vi "Dichtheitstest.vi"() -> ()   [LabVIEW 2020, in "Erweiterte Konfig.lvlib"]
uses:
  Erweiterte Konfig.lvlib
  Visualisierungs Elemente/Button.ctl
  Visualisierungs Elemente/Zahlen-Ausgabefeld.ctl
  Dichtheitstest Umfang.ctl
  Funktionstasten/Freigabe Aktionen.ctl
  PNS/Aktionen FGV Grenzwerte.ctl
  FGV PID Aktionen.ctl
  Aktionen Dichtheitstest.ctl
  Stoerungen/Stoerungen Messgeraet/Aktionen Kommunikation Stoerung.ctl
  Status Dichtheitstest Aktionen.ctl
  Funktionstasten/Funktionstasten-Aktion.ctl
  Funktionstasten/Zustaende.ctl
  Schedule Modul/Aktion FGV Testdaten sammeln.ctl
  Amium PNS/AK Kommunikation/Amium Kommandos verwalten Aktionen.ctl
  SysLog/SysLog Interface.ctl
  Stoerungen/Stoerungen.lvlib
  Funktionstasten/Funktionstasten.lvlib
  Allgemein/allgemeine Sub-VIs.lvlib
  cRIO/PC/Kommunikation mit cRIO.lvlib
  Sprachverwaltung/Sprachverwaltung.lvlib
  SysLog/SysLog.lvlib
  Amium PNS/AK Kommunikation/AK Kommunikation.lvlib
  Auto Kalibrieren/VI Auto Kalibrieren.vi
  Auto Kalibrieren/Auto Kalibrieren.lvlib
  PNS/PNS.lvlib
  Schedule Modul/Schedule Modul.lvlib
  Sprachverwaltung/FGV Aktion Tabelle zerlegen.ctl
panel:
  out "Dichtheitstest Umfang":T1 items=["Pumpe / Filter / FT-IR / PNS", "Pumpe / Filter / FT-IR", "Filter / FT-IR", "FT-IR"]
  out "Status":string
  out "Druckanstieg:":T2
  out "Verstrichene Zeit:":T2
  out "Zeitdauer:":T2
  out "max. Anstieg:":T2 caption="max. Druckanstieg:"
  out "Druck FT-IR:":T2 format="%.3f"
  in  "BEENDEN":T3
  # "Dichtheitstest"
  # "bar"
  # "mbar"
  # "mbar"
  # "sec"
  # "sec"
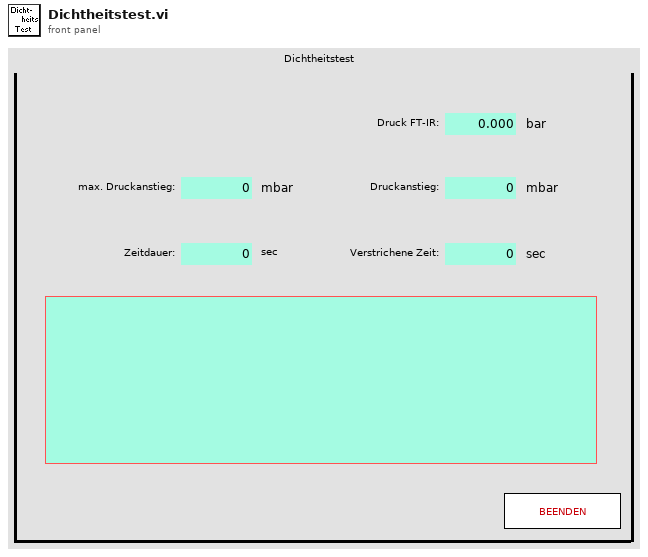
[diagram p1: front panel]
types:
  T1 = typedef "Erweiterte Konfig.lvlib/Dichtheitstest Umfang.ctl" = u16
  T2 = typedef "Zahlen-Ausgabefeld.ctl" = sgl
  T3 = typedef "Button.ctl" = bool
  T4 = typedef "PNS.lvlib/Aktionen FGV Grenzwerte.ctl" = enum16{"lesen", "Grenzw. schreiben", "Anweisungscode", "IP-Adresse", "laden", "speichern", "Anweisungscode vorgeben"}
  T5 = typedef "Funktionstasten.lvlib/Freigabe Aktionen.ctl" = enum16{"prüfen", "Freigabe?", "lesen"}
  T6 = typedef "Erweiterte Konfig.lvlib/Status Dichtheitstest Aktionen.ctl" = enum16{"lesen", "Zeitstempel", "Daten", "läuft", "Protokolldaten"}
  T7 = typedef "Stoerungen.lvlib/Aktionen Kommunikation Stoerung.ctl" = enum16{"lesen", "init", "FT-IR Komm", "FT-IR Betriebsart", "FT-IR Hintergrund", "cRIO Komm", "PNS Komm", "Dichtheitstest", "Life Bit", "FTIR Komm AK", "PMA Komm", "FID Komm", "PMA Cal", "FID Ch4 Cal", "FID THC Cal", "Cal Timeout", "VFS 1 Komm", "VFS 2 Komm", "VFS 3 Komm", "VFS 4 Komm", "TRE 08 Komm", "CG-Test vorzeitig", "CG-Test Span 1", "CG-Test Span 2", "CG-Test Span 3", "CG-Test Messgas", "CG-Test löschen", "Test", "Amium AK", "AK Recept konfig", "AK Name konfig", "AK EKFG konfig"}
  T8 = typedef "Erweiterte Konfig.lvlib/FGV PID Aktionen.ctl" = enum16{"Lesen", "Schreiben PID", "Schreiben Sonstige", "Dichtheitstest", "Aktionen Dicht.", "Parameter Sensor"}
  T9 = typedef "Erweiterte Konfig.lvlib/Aktionen Dichtheitstest.ctl" = enum16{"Initialisieren", "Unterdruck aufbauen", "Prop schließen", "Warten", "Auswertung", "Fertig"}
  T10 = typedef "Steuerung PNS.lvclass/Anlegengrenzwerte PNS.ctl" = cluster{"Filter:":T11, "Ventilplatte:":T11, "Heizleitung 1:":T11, "Heizleitung 2:":T11, "Heizleitung 3:":T11, "Heizleitung 4:":T11, "Heizleitung 5:":T11, "Heizleitung 6:":T11}
  T11 = typedef "Steuerung PNS.lvclass/Anlagengrenzwerte Parameteranzeige.ctl" = cluster{"Sollwert":T12, "Warn-Min":T12, "Warn-Max":T12, "Abschalt-Min":T12, "Abschalt-Max":T12, "Regler":u16, "AnlagenParameter":string}
  T12 = typedef "Zahlen-Eingabefeld.ctl" = sgl
  T13 = typedef "Erweiterte Konfig.lvlib/Sonstige Parameter.ctl" = cluster{"Lüfter langsam":sgl, "Lüfter schnell":sgl, "FT-IR Kühlung Soll":sgl, "FT-IR Kühlung Max":sgl, "Überwachung":T14, "Befüllung aktiv":T15, "Stickstoff Befüllzeit":sgl, "Befüllintervall":sgl, "Kalibrierwert FT-IR":sgl, "Offset Ausgang":sgl, "Offset FT-IR":sgl, "Offset Druck FT-IR":sgl, "Dichtheitstest Zeit":sgl, "Dichtheitstest Abfall":sgl, "Dichtheitstest Umfang":T1, "Offset Umgebung":sgl, "Max Taupunkt":sgl, "Pumpendrehzahl":sgl, "ext. Befüllung":T15, "Ext. Stickstoff Befüllzeit":sgl}
  T14 = typedef "Auswahlfeld.ctl" = u16
  T15 = typedef "LogKonfig.lvlib/Auswahlfeld aktiviert-deaktiviert.ctl" = u16
  T16 = typedef "Verwaltung - cRIO.lvlib/Analog Eingaenge.ctl" = cluster{"AI0: Durchfluss FT-IR":sgl, "AI1: Druck Ausgang":sgl, "AI2: Umgebungsdruck":sgl, "AI3: Druck FT-IR":sgl, "AI4: Druck CalGas":sgl, "AI5: Reserve":sgl, "AI6: Reserve":sgl, "AI7: Reserve":sgl, "Rohwert Durchfluss FT-IR":sgl, "Rohwert Druck Ausgang":sgl, "Rohwert Umgebungsdruck":sgl, "Rohwert Druck FT-IR":sgl, "Rohwert Druck CalGas":sgl, "Rohwert AI5":sgl, "Rohwert AI6":sgl, "Rohwert AI7":sgl, "Rohwert Diffdruck mbar FTIR":sgl}
  T17 = typedef "Erweiterte Konfig.lvlib/Dichtheitstest Protokoll.ctl" = cluster{"Startzeit":timestamp, "Endzeit":timestamp, "Startdruck":sgl, "Enddruck":sgl, "Dichtheitstest Umfang":T1}
  T18 = typedef "Schedule Modul.lvlib/Aktion FGV Testdaten sammeln.ctl" = enum16{"lesen", "Dichtheitstest", "CalGasTest", "T90", "Kalibrieren", "init", "Kalender Daten"}
  T19 = typedef "Funktionstasten.lvlib/Zustaende.ctl" = enum16{"Standby", "Pause", "Eco", "Messen", "Kalibrieren", "Spülen Filter", "Spülen Leitung", "Umgebungsluft", "0-Gas", "Cal-Gas", "CG zu PNS", "-------------", "Init 1", "Init 2", "Init 3", "Init 4", "Messen vorbereiten", "Messen durchführen", "Exit"}
  T20 = typedef "Funktionstasten.lvlib/Funktionstasten-Aktion.ctl" = enum16{"Initialisieren", "Zustand setzen", "Taste gedrückt", "Fehler speichern", "Lesen", "Manuell", "Remote", "Bitparallel", "Samplepoint", "Zeit Prüfen", "reset Umschalten"}
  T21 = typedef "Schedule Modul.lvlib/Ergebnis Dichtheitstest.ctl" = cluster{"Druck FT-IR:":T2, "max. Anstieg:":T2, "Druckanstieg:":T2, "Zeitdauer:":T2, "Verstrichene Zeit:":T2, "Fehler":bool, "Unterdruck nicht erreicht ":bool}
  T22 = typedef "Amium PNS.lvlib/AK Kommunikation.lvlib/Amium Kommandos verwalten Aktionen.ctl" = enum16{"lesen", "setzen Ende", "setzen Pos1", "senden", "initalisieren", "prüfen", "Kommandos"}
  T23 = typedef "Sprachverwaltung.lvlib/FGV Aktion Tabelle zerlegen.ctl" = enum16{"laden", "vereinzeln", "speichern"}
  T24 = typedef "SysLog.lvlib/SysLog Interface.ctl" = cluster{"FehlermeldungsCode":i32, "ErfolgsmeldungsCode":i32, "ParameterListenString":string, "Anzeige":bool, "SysLogIcon":enum16{"OK", "Warnung", "Fehler"}, "intern":bool}
  T25 = typedef "Stoerungen.lvlib/Stoerungen Messgeraete.ctl" = cluster{"FT-IR Komm":bool, "FT-IR Betriebsart":bool, "FT-IR Hintergrundscan":bool, "Dichtheitstest":bool, "cRIO Komm":bool, "PNS Komm":bool, "Life Bit":bool, "FT-IR AK Komm":bool, "PMA Komm":bool, "FID Komm":bool, "PMA Cal":bool, "FID CH4 Cal":bool, "FID THC Cal":bool, "Cal Timeout":bool, "VFS 1 Komm":bool, "VFS 2 Komm":bool, "VFS 3 Komm":bool, "VFS 4 Komm":bool, "TRE 08 Komm":bool, "CG-Test":bool, "CG-Test 1":bool, "CG-Test 2":bool, "CG-Test 3":bool, "Messgas - Eingang":bool, "Amium AK Komm":bool, "AK Rezept nicht konfiguriert ":bool, "AK Name nicht konfiguriert":bool, "AK EKFG nicht konfiguriert":bool}
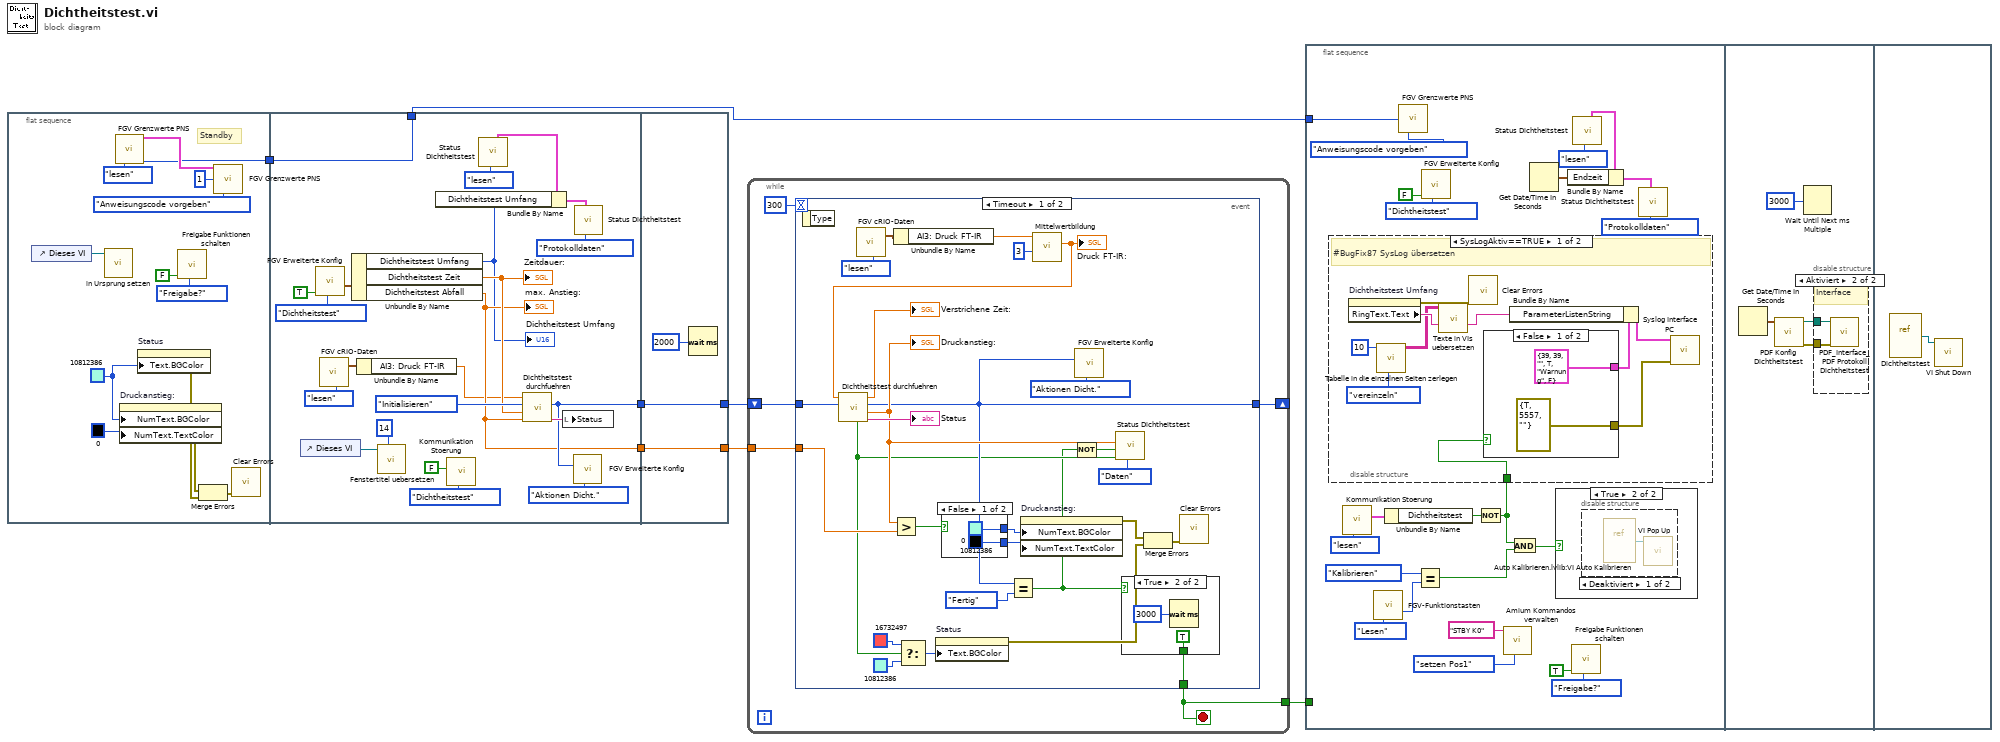
[diagram p0: block diagram]
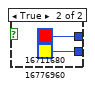
[diagram p3: hidden frame]
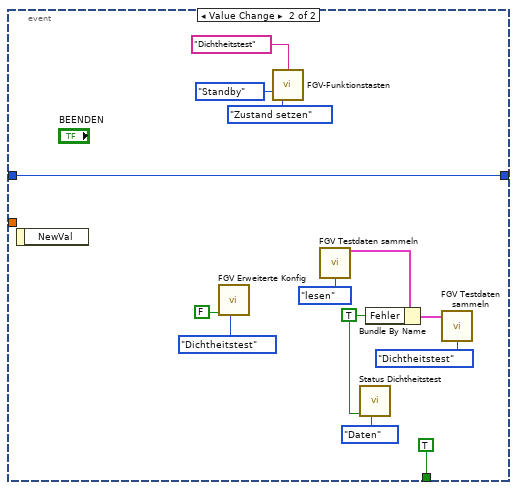
[diagram p4: hidden frame]
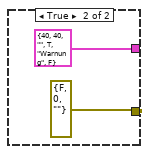
[diagram p5: hidden frame]
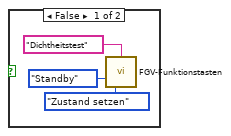
[diagram p7: hidden frame]
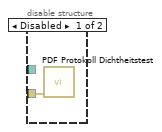
[diagram p9: hidden frame]
diagram:
  n1 = flat-sequence {
    tunnel: [w9] -> w2
    tunnel: [w35] -> w7
    tunnel: [w34] -> w6
    tunnel: w2 -> [w21]
    tunnel: [w21] -> w1
    tunnel: [w45] -> w5
    tunnel: w7 -> [w45]
    tunnel: w6 -> [w43]
    tunnel: [w43] -> w4
    frame #0 {
      w20 = u32 10812386 ("Hintergrund")
      # "Standby"
      n2 = control-ref of="Dieses VI"() -> (w8:refnum<vi>)
      n3 = call "in Ursprung setzen.vi"("VI Referenz"=w8) -> ()  [unwired: 10 in, 1 out]
      n4 = call "FGV Grenzwerte PNS.vi"("Aktionen FGV Grenzwerte"=Aktionen_FGV_Grenzwerte."lesen") -> ("Grenzwerte PNS 2"=w10:T10, "Anweisungscode"=w9:u16)  [unwired: 12 in, 1 out]
      n5 = property on="Druckanstieg:" class="DigWert (strikt)"("NumText.BGColor"=w20, "NumText.TextColor"=u32 0 ("Hintergrund")) -> (error out=w16:errorcluster)  [unwired: 2 in, 1 out]
      n6 = property on="Status" class="Str"("Text.BGColor"=w20) -> (error out=w17:errorcluster)  [unwired: 2 in, 1 out]
      n7 = call "Freigabe Funktionen schalten.vi"("Aktionen"=Freigabe_Aktionen."Freigabe?", "Freigabe?"=FALSE) -> ()  [unwired: 7 in, 3 out]
      n8 = Merge Errors(w16, w17) -> (w18:errorcluster)
      n9 = call "FGV Grenzwerte PNS.vi"("Grenzwerte PNS"=w10, "Anweisungscode"=u16 1, "Aktionen FGV Grenzwerte"=Aktionen_FGV_Grenzwerte."Anweisungscode vorgeben") -> ()  [unwired: 10 in, 3 out]
      n10 = call <vilib>:"Clear Errors.vi"("error in (no error)"=w18) -> ()  [unwired: 5 in, 2 out]
    }
    frame #1 {
      n11 = control-ref of="Dieses VI"() -> (w28:refnum<vi>)
      n12 = call "FGV Erweiterte Konfig.vi"("Aktion"=FGV_PID_Aktionen."Dichtheitstest", "Dichtheitstest?"=TRUE) -> ("Sonstige"=w42:T13)  [unwired: 5 in, 4 out]
      n13 = call "FGV cRIO-Daten.vi"("Aktion"=enum16{"lesen", "schreiben"}."lesen") -> ("Analog Input"=w30:T16)  [unwired: 9 in, 9 out]
      n14 = Unbundle By Name(w42) -> ("Dichtheitstest Umfang"=w22:T1, "Dichtheitstest Zeit"=w38:sgl, "Dichtheitstest Abfall"=w34:sgl)
      "max. Anstieg:" <- w34
      "Zeitdauer:" <- w38
      "Dichtheitstest Umfang" <- w22
      n15 = Unbundle By Name(w30) -> ("AI3: Druck FT-IR"=w29:sgl)
      n16 = call "Fenstertitel uebersetzen.vi"("Index (Seite)"=14, "Dieses VI"=w28) -> ()  [unwired: 6 in, 4 out]
      n17 = call "Kommunikation Stoerung.vi"("Aktionen"=Aktionen_Kommunikation_Stoerung."Dichtheitstest", "ERROR"=FALSE) -> ()  [unwired: 9 in, 1 out]
      n18 = call "Status Dichtheitstest.vi"("Aktionen"=Status_Dichtheitstest_Aktionen."lesen") -> ("Protokoll"=w25:T17)  [unwired: 6 in, 4 out]
      n19 = Bundle By Name(cluster=w25, "Dichtheitstest Umfang"=w22) -> (w26:T17)
      n20 = call "Dichtheitstest durchfuehren.vi"("max. Druckanstieg"=w34, "Wartezeit"=w38, "Aktionen"=Aktionen_Dichtheitstest."Initialisieren", "Druck FT-IR"=w29) -> ("Status"=w37:string, "Aktionen"=w35:T9)  [unwired: 3 in, 3 out]
      n21 = local write "Status"(w37) -> ()
      n22 = call "FGV Erweiterte Konfig.vi"("Aktion"=FGV_PID_Aktionen."Aktionen Dicht.", "Aktionen Dichtheitstest"=w35) -> ()  [unwired: 5 in, 5 out]
      n23 = call "Status Dichtheitstest.vi"("Aktionen"=Status_Dichtheitstest_Aktionen."Protokolldaten", "Protokoll"=w26) -> ()  [unwired: 5 in, 5 out]
    }
    frame #2 {
      n24 = Wait (ms)(milliseconds to wait=u32 2000 ("Zu wartende ms")) -> ()  [unwired: 1 out]
    }
  }
  n25 = while {
    shift-right: [w48] -> _
    shift-left: w5 -> [w49]
    tunnel: w4 -> [w47]
    tunnel: [w46] -> w3
    stop <- w46 stop-if-true
    n26 = event shown="[0] Timeout" {
      selector: _ -> [_ _]
      dyn-events: _ -> [_ _]
      timeout: 300 -> [_ _]
      tunnel: [w65 TRUE ("ABBRECHEN")] -> w46
      tunnel: w49 -> [w77 w96]
      tunnel: [w54 w96] -> w48
      tunnel: w47 -> [w73 _]
      event Timeout {
        n27 = event-data() -> ()  [unwired: 1 in, 1 out]
        n28 = call "FGV cRIO-Daten.vi"("Aktion"=enum16{"lesen", "schreiben"}."lesen") -> ("Analog Input"=w64:T16)  [unwired: 9 in, 9 out]
        n29 = Unbundle By Name(w64) -> ("AI3: Druck FT-IR"=w61:sgl)
        n30 = call "Mittelwertbildung.vi"("Anzahl Werte"=u8 3, "Neuer Wert"=w61) -> ("gemittelter Wert"=w60:sgl)  [unwired: 7 in, 2 out]
        "Druck FT-IR:" <- w60
        n31 = call "Dichtheitstest durchfuehren.vi"("Aktionen"=w77, "Druck FT-IR"=w60) -> ("Status"=→"Status":string, "Druckabfall"=w55:sgl, "Aktionen"=w54:T9, "Verstrichene Zeit"=→"Verstrichene Zeit:":sgl, "Fehler"=w53:bool)  [unwired: 5 in]
        "Druckanstieg:" <- w55
        n32 = Greater?(x=w55, y=w73) -> (0:w67:bool)
        n33 = Select(t=u32 16732497 ("Hintergrund"), s=w53, f=u32 10812386 ("Hintergrund")) -> (s? t:f=w68:u32)
        n34 = property on="Status" class="Str"("Text.BGColor"=w68) -> (error out=w59:errorcluster)  [unwired: 2 in, 1 out]
        n35 = case shown="False" w67 {
          tunnel: [u32 10812386 ("Hintergrund") u32 16711680 ("Hintergrund")] -> w71
          tunnel: [u32 0 ("Hintergrund") u32 16776960 ("Hintergrund")] -> w72
          frame False {
          }
          frame True {
          }
        }
        n36 = Equal?(x=w54, y=Aktionen_Dichtheitstest."Fertig") -> (x = y?=w51:bool)
        n37 = property on="Druckanstieg:" class="DigWert (strikt)"("NumText.BGColor"=w71, "NumText.TextColor"=w72) -> (error out=w58:errorcluster)  [unwired: 2 in, 1 out]
        n38 = Not(x=w51) -> (.not. x?=w52:bool)
        n39 = call "FGV Erweiterte Konfig.vi"("Aktion"=FGV_PID_Aktionen."Aktionen Dicht.", "Aktionen Dichtheitstest"=w54) -> ()  [unwired: 5 in, 5 out]
        n40 = call "Status Dichtheitstest.vi"("Aktionen"=Status_Dichtheitstest_Aktionen."Daten", "Fehler"=w53, "läuft?"=w52, "Anstieg"=w55) -> ()  [unwired: 3 in, 5 out]
        n41 = case shown="True" w51 {
          tunnel: [_ TRUE] -> w65
          frame False {
          }
          frame True {
            n42 = Wait (ms)(milliseconds to wait=u32 3000 ("Zu wartende ms")) -> ()  [unwired: 1 out]
          }
        }
        n43 = Merge Errors(w58, w59) -> (w57:errorcluster)
        n44 = call <vilib>:"Clear Errors.vi"("error in (no error)"=w57) -> ()  [unwired: 5 in, 2 out]
      }
      event Value Change {
        w84 = TRUE ("Fehler")
        n45 = event-data() -> ()  [unwired: 1 in, 1 out]
        n46 = call "FGV Erweiterte Konfig.vi"("Aktion"=FGV_PID_Aktionen."Dichtheitstest", "Dichtheitstest?"=FALSE) -> ()  [unwired: 5 in, 5 out]
        n47 = call "FGV-Funktionstasten.vi"("Herkunft"="Dichtheitstest", "Zustand"=Zustaende."Standby", "Aktion"=Funktionstasten-Aktion."Zustand setzen") -> ()  [unwired: 5 in, 8 out]
        n48 = call "FGV Testdaten sammeln.vi"("Aktion"=Aktion_FGV_Testdaten_sammeln."lesen") -> ("Ergebnisse Dichtheitstest"=w86:T21)  [unwired: 9 in, 5 out]
        n49 = call "Status Dichtheitstest.vi"("Aktionen"=Status_Dichtheitstest_Aktionen."Daten", "Fehler"=w84) -> ()  [unwired: 5 in, 5 out]
        n50 = Bundle By Name(cluster=w86, "Fehler"=w84) -> (w87:T21)
        n51 = call "FGV Testdaten sammeln.vi"("Ergebnisse Dichtheitstest"=w87, "Aktion"=Aktion_FGV_Testdaten_sammeln."Dichtheitstest") -> ()  [unwired: 8 in, 6 out]
      }
    }
  }
  n52 = flat-sequence {
    tunnel: w3 -> [_]
    tunnel: w1 -> [w97]
    frame #0 {
      n53 = call "Kommunikation Stoerung.vi"("Aktionen"=Aktionen_Kommunikation_Stoerung."lesen") -> ("Störung Messgerät"=w113:T25)  [unwired: 10 in]
      n54 = call "FGV-Funktionstasten.vi"("Aktion"=Funktionstasten-Aktion."Lesen") -> ("ausgewählte Funktion"=w115:T19)  [unwired: 7 in, 7 out]
      n55 = Unbundle By Name(w113) -> ("Dichtheitstest"=w117:bool)
      n56 = call "FGV Grenzwerte PNS.vi"("Anweisungscode"=w97, "Aktionen FGV Grenzwerte"=Aktionen_FGV_Grenzwerte."Anweisungscode vorgeben") -> ()  [unwired: 11 in, 3 out]
      n57 = Equal?(x=Zustaende."Kalibrieren", y=w115) -> (x = y?=w118:bool)
      n58 = call "FGV Erweiterte Konfig.vi"("Aktion"=FGV_PID_Aktionen."Dichtheitstest", "Dichtheitstest?"=FALSE) -> ()  [unwired: 5 in, 5 out]
      n59 = Not(x=w117) -> (.not. x?=w108:bool)
      n60 = disable-structure shown="SysLogAktiv==TRUE" {
        disable-tunnel: w108 -> [w128 _]
        frame condition #0 (active) {
          # "#BugFix87 SysLog übersetzen"
          n61 = property on="Dichtheitstest Umfang" class="Ring (strikt)"() -> (error out=w126:errorcluster, "RingText.Text"=w123:string)  [unwired: 2 in, 1 out]
          n62 = call "Tabelle in die einzelnen Seiten zerlegen.vi"("Aktion"=FGV_Aktion_Tabelle_zerlegen."vereinzeln", "Index (Seite)"=10) -> ("Sprachliste"=w119:string[][])  [unwired: 7 in, 2 out]
          n63 = call "Texte in VIs uebersetzen.vi"("Sprachliste"=w119, "String zum Übersetzen"=w123) -> ("String zum Übersetzen"=w122:string)  [unwired: 9 in, 4 out]
          n64 = call <vilib>:"Clear Errors.vi"("error in (no error)"=w126) -> ()  [unwired: 5 in, 2 out]
          n65 = case shown="False" w128 {
            tunnel: [errorcluster {"status"=TRUE, "code"=5557, "source"=""} ("Fehler (in)") errorcluster {"status"=FALSE, "code"=0, "source"=""} ("Fehler (in)")] -> w127
            tunnel: [T24 {"FehlermeldungsCode"=39, "ErfolgsmeldungsCode"=39, "ParameterListenString"="", "Anzeige"=TRUE, "SysLogIcon"=enum."Warnung", "intern"=FALSE} ("Cluster (in)") T24 {"FehlermeldungsCode"=40, "ErfolgsmeldungsCode"=40, "ParameterListenString"="", "Anzeige"=TRUE, "SysLogIcon"=enum."Warnung", "intern"=FALSE} ("Cluster (in)")] -> w125
            frame False {
            }
            frame True {
            }
          }
          n66 = Bundle By Name(cluster=w125, "ParameterListenString"=w122) -> (w124:T24)
          n67 = call "Syslog Interface PC.vi"("Fehler (in)"=w127, "Cluster (in)"=w124) -> ()  [unwired: 9 in, 1 out]
        }
        frame condition #1 {
        }
      }
      n68 = call "Amium Kommandos verwalten.vi"("Aktionen"=Amium_Kommandos_verwalten_Aktionen."setzen Pos1", "neues Kommando"="STBY K0") -> ()  [unwired: 7 in, 3 out]
      n69 = And(x=w108, y=w118) -> (x .and. y?=w111:bool)
      n70 = Get Date/Time In Seconds() -> (seconds since 1Jan1904=w101:timestamp)
      n71 = case shown="True" w111 {
        frame False {
          n72 = call "FGV-Funktionstasten.vi"("Herkunft"="Dichtheitstest", "Zustand"=Zustaende."Standby", "Aktion"=Funktionstasten-Aktion."Zustand setzen") -> ()  [unwired: 5 in, 8 out]
        }
        frame True {
          n73 = disable-structure shown="Deaktiviert" {
            frame Disabled {
              n74 = vi-ref "Auto Kalibrieren.lvlib:VI Auto Kalibrieren.vi"() -> (w136:refnum<vi>)
              n75 = call "VI Pop Up.vi"("VI Referenz"=w136) -> ()  [unwired: 10 in, 1 out]
            }
            frame Enabled {
            }
          }
        }
      }
      n76 = call "Freigabe Funktionen schalten.vi"("Aktionen"=Freigabe_Aktionen."Freigabe?", "Freigabe?"=TRUE) -> ()  [unwired: 7 in, 3 out]
      n77 = call "Status Dichtheitstest.vi"("Aktionen"=Status_Dichtheitstest_Aktionen."lesen") -> ("Protokoll"=w102:T17)  [unwired: 6 in, 4 out]
      n78 = Bundle By Name(cluster=w102, "Endzeit"=w101) -> (w105:T17)
      n79 = call "Status Dichtheitstest.vi"("Aktionen"=Status_Dichtheitstest_Aktionen."Protokolldaten", "Protokoll"=w105) -> ()  [unwired: 5 in, 5 out]
    }
    frame #1 {
      n80 = Get Date/Time In Seconds() -> (seconds since 1Jan1904=w139:timestamp)
      n81 = call "PDF Konfig Dichtheitstest.vi"("seconds since 1Jan1904"=w139) -> ("error out"=w140:errorcluster, "PDF Pfad"=w137:path)  [unwired: 9 in]
      n82 = Wait Until Next ms Multiple(millisecond multiple=u32 3000 ("ms")) -> ()  [unwired: 1 out]
      n83 = disable-structure shown="Aktiviert" {
        disable-tunnel: w140 -> [w141 w143]
        disable-tunnel: w137 -> [_ w142]
        frame Disabled {
          n84 = call "PDF Protokoll Dichtheitstest.vi"("error in (no error)"=w141) -> ()  [unwired: 10 in, 1 out]
        }
        frame Enabled {
          # "#PDF_Interface"
          n85 = call "PDF_Interface_PDF Protokoll Dichtheitstest.vi"("error in (no error)"=w143, "Save PDF File Path"=w142) -> ()  [unwired: 9 in, 1 out]
        }
      }
    }
    frame #2 {
      n86 = vi-ref "Dichtheitstest.vi"() -> (w144:refnum<vi>)
      n87 = call "VI Shut Down.vi"("VI Referenz"=w144) -> ()  [unwired: 11 in]
    }
  }
